vi "Write.vi"(8 "error in (no error)":errorcluster, 10 "Enum Variant":variant, 11 "Enum in":refnum<class "Enum.lvclass">) -> (0 "error out":errorcluster, 1 "Success?":bool, 3 "Enum out":refnum<class "Enum.lvclass">)   [LabVIEW 2020, in "Data.lvlib" / "Enum.lvclass"]
doc: "Write Enum."
uses:
  Enum.lvclass
  Enum.lvclass/Enum.ctl
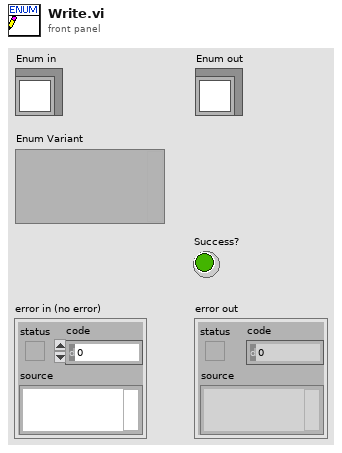
[diagram p1: front panel]
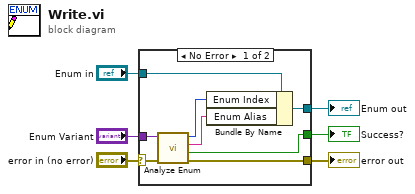
[diagram p0: block diagram]
diagram:
  n1 = case shown="No Error" "error in (no error)" {
    selector: "error in (no error)" -> [w13 w15]
    tunnel: [w14 w15] -> w5
    tunnel: [w7 w16] -> w3
    tunnel: "Enum in" -> [w8 w16]
    tunnel: "Enum Variant" -> [w12 _]
    tunnel: [w11 _] -> w1
    frame No Error {
      n2 = call "Analyze Enum.vi"("error in (no error)"=w13, "Enum Variant"=w12) -> ("error dub"=w14:errorcluster, "Success?"=w11:bool, "Enum Alias"=w9:string, "Enum Index"=w10:u32)  [unwired: 6 in]
      n3 = Bundle By Name(cluster=w8, "Enum Index"=w10, "Enum Alias"=w9) -> (w7:refnum<class "Enum.lvclass">)
    }
    frame Error {
    }
  }
  "error out" <- w5
  "Enum out" <- w3
  "Success?" <- w1
